vi "Mark_GetMarkVar.vi"(8 "error in (no error)":errorcluster, 9 "VarIdx(0)":i32, 10 "VarName":string, 11 "ExpData in":refnum<class "ExpData.lvclass">) -> (0 "error out":errorcluster, 1 "Var":dbl[](graph), 2 "Time":dbl[](array[numeric]), 3 "ExpData out":refnum<class "ExpData.lvclass">, 4 "Var_All":dbl[][](array[numeric]))   [LabVIEW 2016, in "ExpData.lvclass"]
uses:
  ExpData.lvclass
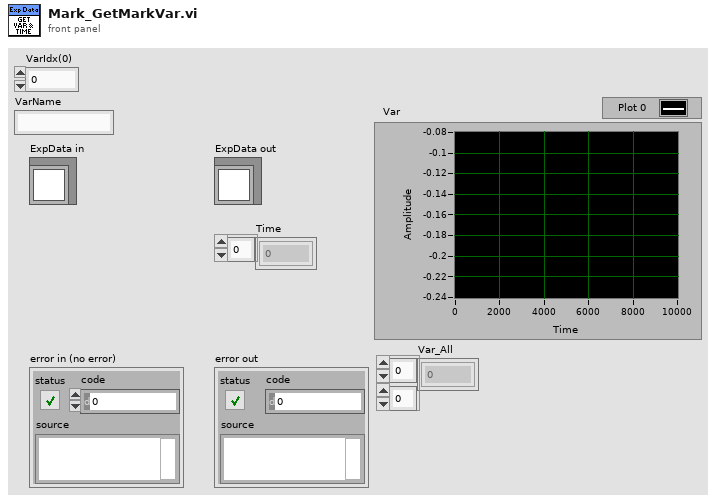
[diagram p1: front panel]
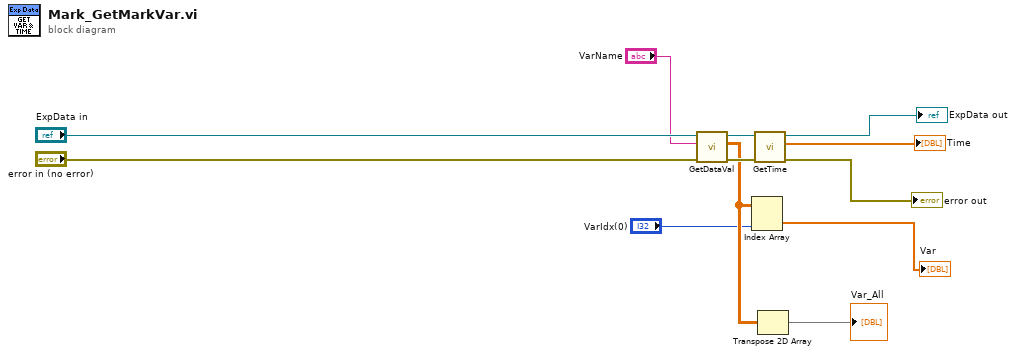
[diagram p0: block diagram]
diagram:
  n1 = call "GetDataVal.vi"("error in (no error)"="error in (no error)", "Name"="VarName", "CarexMData in"="ExpData in") -> ("error out"=w6:errorcluster, "Data"=w4:dbl[][], "CarexMData out"=w5:refnum<class "ExpData.lvclass">)  [unwired: 5 in, 1 out]
  n2 = Index Array(array=w4, index (col)="VarIdx(0)") -> (element=→"Var":dbl[])  [unwired: 1 in]
  n3 = call "GetTime.vi"("error in (no error)"=w6, "CarexMData in"=w5) -> ("error out"=→"error out":errorcluster, "Time"=→"Time":dbl[], "CarexMData out"=→"ExpData out":refnum<class "ExpData.lvclass">)  [unwired: 7 in]
  n4 = Transpose 2D Array(2D array=w4) -> (transposed array=→"Var_All":dbl[][])
